vi "USB2CANFD_Test.vi"() -> ()   [LabVIEW 2010]
panel:
  in  "SpeedBpsDBT":u32(ring)=2000000 items=["5000 Kbps"=5000000, "2000 Kbps"=2000000, "1000 Kbps"=1000000, "500 Kbps"=500000, "250 Kbps"=250000, "200 Kbps"=200000, "125 Kbps"=125000, "100 Kbps"=100000, ""=0]
  in  "SpeedBpsNBT":u32(ring)=500000 items=["1000 Kbps"=1000000, "500 Kbps"=500000, "250 Kbps"=250000, "200 Kbps"=200000, "125 Kbps"=125000, "100 Kbps"=100000, ""=0]
  in  "Receive Channel":u8(ring)=1 items=["CAN1", "CAN2"]
  in  "Send Channel":u8(ring) items=["CAN1", "CAN2"]
  out "Get Msg Num":i32
  out "pCanGetMsg OUT":T1(array[cluster])
  in  "stop":bool
  out "Success Sended Msg Num":i32
  in  "pCanSendMsg":T2={"ID"=1, "DLC"=8, "Flags"=0, "__Res0"=0, "__Res1"=0, "TimeStamp"=0, "Data[0]"=1, "Data[1]"=2, "Data[2]"=3, "Data[3]"=4, "Data[4]"=5, "Data[5]"=6, "Data[6]"=7, "Data[7]"=8, "Data[8]"=0, "Data[9]"=0, "Data[10]"=0, "Data[11]"=0, "Data[12]"=0, "Data[13]"=0, "Data[14]"=0, "Data[15]"=0, "Data[16]"=0, "Data[17]"=0, "Data[18]"=0, "Data[19]"=0, "Data[20]"=0, "Data[21]"=0, "Data[22]"=0, "Data[23]"=0, "Data[24]"=0, "Data[25]"=0, "Data[26]"=0, "Data[27]"=0, "Data[28]"=0, "Data[29]"=0, "Data[30]"=0, "Data[31]"=0, "Data[32]"=0, "Data[33]"=0, "Data[34]"=0, "Data[35]"=0, "Data[36]"=0, "Data[37]"=0, "Data[38]"=0, "Data[39]"=0, "Data[40]"=0, "Data[41]"=0, "Data[42]"=0, "Data[43]"=0, "Data[44]"=0, "Data[45]"=0, "Data[46]"=0, "Data[47]"=0, "Data[48]"=0, "Data[49]"=0, "Data[50]"=0, "Data[51]"=0, "Data[52]"=0, "Data[53]"=0, "Data[54]"=0, "Data[55]"=0, "Data[56]"=0, "Data[57]"=0, "Data[58]"=0, "Data[59]"=0, "Data[60]"=0, "Data[61]"=0, "Data[62]"=0, "Data[63]"=0} {"ID" format="%x"; "Data[1]" format="%x"; "Data[2]" format="%x"}
  in  "Device Index":i32(ring) items=["0", "1", "2", "3", "4", "5"]
  in  "pCanGetMsg":T2
  in  "pCanConfig":T3={"Mode"=0, "ISOCRCEnable"=1, "RetrySend"=3, "ResEnable"=1, "NBT_BRP"=1, "NBT_SEG1"=59, "NBT_SEG2"=20, "NBT_SJW"=2, "DBT_BRP"=1, "DBT_SEG1"=14, "DBT_SEG2"=5, "DBT_SJW"=2, "__Res0[0]"=0, "__Res0[1]"=0, "__Res0[2]"=0, "__Res0[3]"=0, "__Res0[4]"=0, "__Res0[5]"=0, "__Res0[6]"=0, "__Res0[7]"=0}
  # "测试之前将CAN1和CAN2对接，也就是CAN1的H接CAN2的H，CAN1的L接CAN2的L，CAN1发送数据，CAN2接收数据"
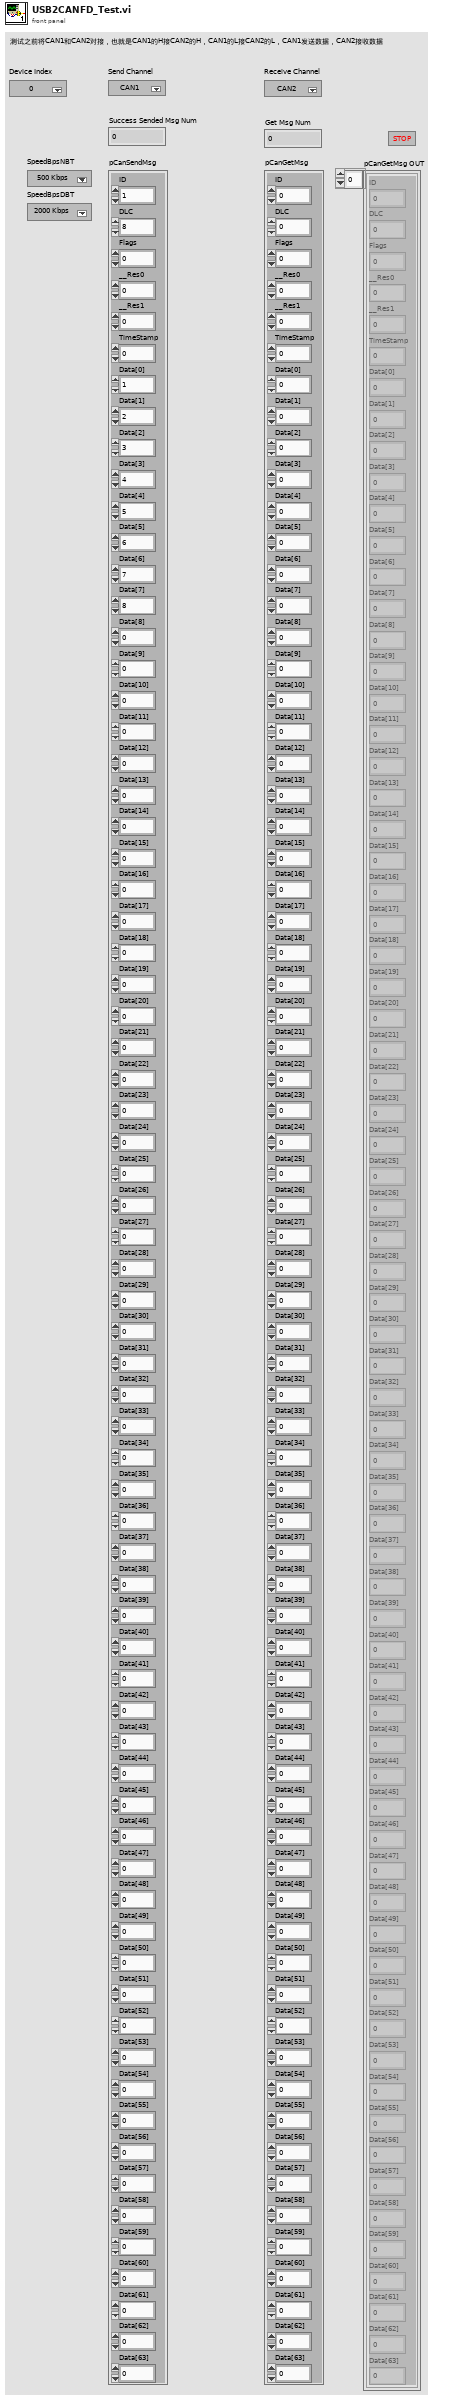
[diagram p1: front panel]
types:
  T1 = cluster{"ID":u32, "DLC":u8, "Flags":u8, "__Res0":u8, "__Res1":u8, "TimeStamp":u32, "Data[0]":u8, "Data[1]":u8, "Data[2]":u8, "Data[3]":u8, "Data[4]":u8, "Data[5]":u8, "Data[6]":u8, "Data[7]":u8, "Data[8]":u8, "Data[9]":u8, "Data[10]":u8, "Data[11]":u8, "Data[12]":u8, "Data[13]":u8, "Data[14]":u8, "Data[15]":u8, "Data[16]":u8, "Data[17]":u8, "Data[18]":u8, "Data[19]":u8, "Data[20]":u8, "Data[21]":u8, "Data[22]":u8, "Data[23]":u8, "Data[24]":u8, "Data[25]":u8, "Data[26]":u8, "Data[27]":u8, "Data[28]":u8, "Data[29]":u8, "Data[30]":u8, "Data[31]":u8, "Data[32]":u8, "Data[33]":u8, "Data[34]":u8, "Data[35]":u8, "Data[36]":u8, "Data[37]":u8, "Data[38]":u8, "Data[39]":u8, "Data[40]":u8, "Data[41]":u8, "Data[42]":u8, "Data[43]":u8, "Data[44]":u8, "Data[45]":u8, "Data[46]":u8, "Data[47]":u8, "Data[48]":u8, "Data[49]":u8, "Data[50]":u8, "Data[51]":u8, "Data[52]":u8, "Data[53]":u8, "Data[54]":u8, "Data[55]":u8, "Data[56]":u8, "Data[57]":u8, "Data[58]":u8, "Data[59]":u8, "Data[60]":u8, "Data[61]":u8, "Data[62]":u8, "Data[63]":u8}[]
  T2 = cluster{"ID":u32, "DLC":u8, "Flags":u8, "__Res0":u8, "__Res1":u8, "TimeStamp":u32, "Data[0]":u8, "Data[1]":u8, "Data[2]":u8, "Data[3]":u8, "Data[4]":u8, "Data[5]":u8, "Data[6]":u8, "Data[7]":u8, "Data[8]":u8, "Data[9]":u8, "Data[10]":u8, "Data[11]":u8, "Data[12]":u8, "Data[13]":u8, "Data[14]":u8, "Data[15]":u8, "Data[16]":u8, "Data[17]":u8, "Data[18]":u8, "Data[19]":u8, "Data[20]":u8, "Data[21]":u8, "Data[22]":u8, "Data[23]":u8, "Data[24]":u8, "Data[25]":u8, "Data[26]":u8, "Data[27]":u8, "Data[28]":u8, "Data[29]":u8, "Data[30]":u8, "Data[31]":u8, "Data[32]":u8, "Data[33]":u8, "Data[34]":u8, "Data[35]":u8, "Data[36]":u8, "Data[37]":u8, "Data[38]":u8, "Data[39]":u8, "Data[40]":u8, "Data[41]":u8, "Data[42]":u8, "Data[43]":u8, "Data[44]":u8, "Data[45]":u8, "Data[46]":u8, "Data[47]":u8, "Data[48]":u8, "Data[49]":u8, "Data[50]":u8, "Data[51]":u8, "Data[52]":u8, "Data[53]":u8, "Data[54]":u8, "Data[55]":u8, "Data[56]":u8, "Data[57]":u8, "Data[58]":u8, "Data[59]":u8, "Data[60]":u8, "Data[61]":u8, "Data[62]":u8, "Data[63]":u8}
  T3 = cluster{"Mode":u8, "ISOCRCEnable":u8, "RetrySend":u8, "ResEnable":u8, "NBT_BRP":u8, "NBT_SEG1":u8, "NBT_SEG2":u8, "NBT_SJW":u8, "DBT_BRP":u8, "DBT_SEG1":u8, "DBT_SEG2":u8, "DBT_SJW":u8, "__Res0[0]":u8, "__Res0[1]":u8, "__Res0[2]":u8, "__Res0[3]":u8, "__Res0[4]":u8, "__Res0[5]":u8, "__Res0[6]":u8, "__Res0[7]":u8}
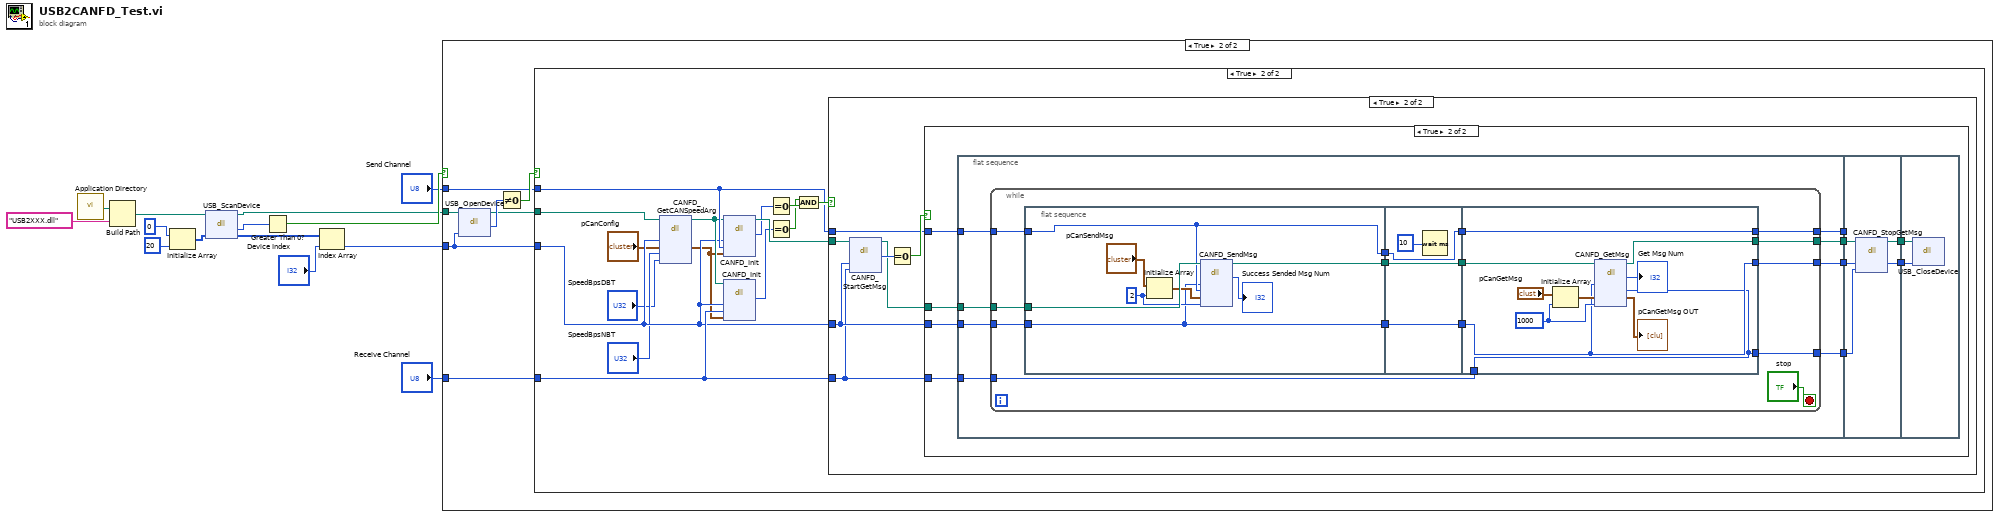
[diagram p0: block diagram]
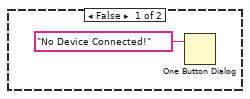
[diagram p2: hidden frame]
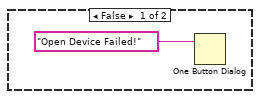
[diagram p3: hidden frame]
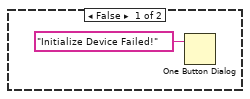
[diagram p4: hidden frame]
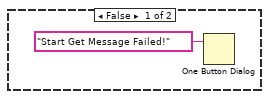
[diagram p5: hidden frame]
diagram:
  n1 = call <vilib>:"Application Directory.vi"() -> ("Application Directory"=w3:path)
  n2 = Build Path(base path=w3, name or relative path="USB2XXX.dll") -> (appended path=w2:path)
  n3 = Initialize Array(0, 20 ("dimension size")) -> (w14:i32[])
  n4 = dll-call lib="E:/OtherWork/STM32/USB2XXX_Example/sdk/api/Labview/USB2XXX.dll" fn="USB_ScanDevice"(path in=w2, "pDevNum"=w14) -> (path out=w6:path, "return type"=w10:i32, "pDevNum"=w11:i32[])  [unwired: 2 in, 1 out]
  n5 = Greater Than 0?(x=w10) -> (x > 0?=w9:bool)
  n6 = Index Array(array=w11, index="Device Index") -> (element=w7:i32)
  n7 = case shown="True" w9 {
    tunnel: w7 -> [_ w19]
    tunnel: w6 -> [_ w20]
    tunnel: "Send Channel" -> [_ w18]
    tunnel: "Receive Channel" -> [_ w16]
    frame False {
      n8 = One Button Dialog(message="No Device Connected!") -> ()  [unwired: 1 in, 1 out]
    }
    frame True {
      n9 = dll-call lib="E:/OtherWork/STM32/USB2XXX_Example/sdk/api/Labview/USB2XXX.*" fn="USB_OpenDevice"(path in=w20, "DevHandle"=w19) -> (path out=w17:path, "return type"=w22:u8)  [unwired: 3 in, 1 out]
      n10 = Not Equal To 0?(x=w22) -> (x != 0?=w21:bool)
      n11 = case shown="True" w21 {
        tunnel: w17 -> [_ w30]
        tunnel: w19 -> [_ w28]
        tunnel: w18 -> [_ w32]
        tunnel: w16 -> [_ w31]
        frame False {
          n12 = One Button Dialog(message="Open Device Failed!") -> ()  [unwired: 1 in, 1 out]
        }
        frame True {
          n13 = dll-call lib="E:/Projects/USB2XXX/trunk/USB2XXX/USB2XXX/vs2019/Release/USB2XXX.*" fn="CANFD_GetCANSpeedArg"(path in=w30, "DevHandle"=w28, "pCanConfig"="pCanConfig", "SpeedBpsNBT"="SpeedBpsNBT", "SpeedBpsDBT"="SpeedBpsDBT") -> (path out=w29:path, "pCanConfig"=w26:T3)  [unwired: 6 in, 1 out]
          n14 = dll-call lib="E:/OtherWork/STM32/USB2XXX_Example/sdk/api/Labview/USB2XXX.*" fn="CANFD_Init"(path in=w29, "DevHandle"=w28, "CANIndex"=w32, "pCanConfig"=w26) -> (path out=w38:path, "return type"=w35:i32)  [unwired: 5 in, 1 out]
          n15 = dll-call lib="E:/OtherWork/STM32/USB2XXX_Example/sdk/api/Labview/USB2XXX.*" fn="CANFD_Init"(path in=w29, "DevHandle"=w28, "CANIndex"=w31, "pCanConfig"=w26) -> ("return type"=w33:i32)  [unwired: 5 in, 2 out]
          n16 = Equal To 0?(x=w35) -> (x = 0?=w37:bool)
          n17 = Equal To 0?(x=w33) -> (x = 0?=w36:bool)
          n18 = And(x=w36, y=w37) -> (x .and. y?=w34:bool)
          n19 = case shown="True" w34 {
            tunnel: w38 -> [_ w46]
            tunnel: w28 -> [_ w41]
            tunnel: w32 -> [_ w42]
            tunnel: w31 -> [_ w40]
            frame False {
              n20 = One Button Dialog(message="Initialize Device Failed!") -> ()  [unwired: 1 in, 1 out]
            }
            frame True {
              n21 = dll-call lib="E:/OtherWork/STM32/USB2XXX_Example/sdk/api/Labview/USB2XXX.*" fn="CANFD_StartGetMsg"(path in=w46, "DevHandle"=w41, "CANIndex"=w40) -> (path out=w43:path, "return type"=w45:i32)  [unwired: 4 in, 1 out]
              n22 = Equal To 0?(x=w45) -> (x = 0?=w44:bool)
              n23 = case shown="True" w44 {
                tunnel: w43 -> [_ w57]
                tunnel: w42 -> [_ w56]
                tunnel: w41 -> [_ w55]
                tunnel: w40 -> [_ w51]
                frame False {
                  n24 = One Button Dialog(message="Start Get Message Failed!") -> ()  [unwired: 1 in, 1 out]
                }
                frame True {
                  n25 = flat-sequence {
                    tunnel: w57 -> [w65]
                    tunnel: w56 -> [w64]
                    tunnel: w55 -> [w63]
                    tunnel: [w62] -> w54
                    tunnel: [w61] -> w53
                    tunnel: [w60] -> w52
                    tunnel: w51 -> [w59]
                    tunnel: [w58] -> w50
                    tunnel: w54 -> [w107]
                    tunnel: w53 -> [w106]
                    tunnel: w52 -> [_]
                    tunnel: w50 -> [w105]
                    tunnel: [w104] -> w49
                    tunnel: [w103] -> w48
                    tunnel: w49 -> [w109]
                    tunnel: w48 -> [w108]
                    frame #0 {
                      n26 = while {
                        tunnel: w65 -> [w80]
                        tunnel: w64 -> [w79]
                        tunnel: w63 -> [w78]
                        tunnel: [w70] -> w62
                        tunnel: [w69] -> w61
                        tunnel: [w68] -> w60
                        tunnel: w59 -> [w67]
                        tunnel: [w66] -> w58
                        stop <- "stop" stop-if-true
                        n27 = flat-sequence {
                          tunnel: w80 -> [w88]
                          tunnel: w79 -> [w83]
                          tunnel: w78 -> [w82]
                          tunnel: [w83] -> w76
                          tunnel: [w82] -> w74
                          tunnel: [w81] -> w72
                          tunnel: w76 -> [w91]
                          tunnel: [w91] -> w75
                          tunnel: w74 -> [w90]
                          tunnel: [w90] -> w73
                          tunnel: w72 -> [w89]
                          tunnel: [w89] -> w71
                          tunnel: w75 -> [w94]
                          tunnel: w73 -> [w95]
                          tunnel: w71 -> [w99]
                          tunnel: [w96] -> w70
                          tunnel: [w95] -> w69
                          tunnel: [w94] -> w68
                          tunnel: w67 -> [w93]
                          tunnel: [w93] -> w66
                          frame #0 {
                            w85 = 2 ("dimension size")
                            n28 = Initialize Array("pCanSendMsg", w85) -> (w86:T1)
                            n29 = dll-call lib="E:/OtherWork/STM32/USB2XXX_Example/sdk/api/Labview/USB2XXX.*" fn="CANFD_SendMsg"(path in=w88, "DevHandle"=w82, "CANIndex"=w83, "pCanSendMsg"=w86, "SendMsgNum"=w85) -> (path out=w81:path, "return type"=→"Success Sended Msg Num":i32)  [unwired: 6 in, 1 out]
                          }
                          frame #1 {
                            n30 = Wait (ms)(milliseconds to wait=u32 10 ("等待时间（毫秒）")) -> ()  [unwired: 1 out]
                          }
                          frame #2 {
                            w100 = 1000 ("BufferSize")
                            n31 = Initialize Array("pCanGetMsg", w100) -> (w101:T1)
                            n32 = dll-call lib="E:/OtherWork/STM32/USB2XXX_Example/sdk/api/Labview/USB2XXX.dll" fn="CANFD_GetMsg"(path in=w99, "DevHandle"=w95, "CANIndex"=w93, "pCanGetMsg"=w101, "BufferSize"=w100) -> (path out=w96:path, "return type"=→"Get Msg Num":i32, "pCanGetMsg"=→"pCanGetMsg OUT":T1)  [unwired: 5 in, 1 out]
                          }
                        }
                      }
                    }
                    frame #1 {
                      n33 = dll-call lib="E:/OtherWork/STM32/USB2XXX_Example/sdk/api/Labview/USB2XXX.*" fn="CANFD_StopGetMsg"(path in=w107, "DevHandle"=w106, "CANIndex"=w105) -> (path out=w104:path, "DevHandle"=w103:i32)  [unwired: 4 in, 1 out]
                    }
                    frame #2 {
                      n34 = dll-call lib="E:/Projects/USB2XXX/trunk/USB2XXX/USB2XXX/vs2010/Release/USB2XXX.*" fn="USB_CloseDevice"(path in=w109, "DevHandle"=w108) -> ()  [unwired: 4 in, 2 out]
                    }
                  }
                }
              }
            }
          }
        }
      }
    }
  }
